vi "HandsOnEmulatedHardware.vi"() -> ()   [LabVIEW 2024]
doc: "DESCRIPTION\nHands On Emulated VISA Hardware\n\nVERSION\nD1:04\nDIs are inverted when compared to hardware - corrected\nRemoved Obsolete GET and SET commands\n20 Oct 2023\n\nD1:03\nMade compatible with CTI-VISA - PWM still to do \n13 Sept 2023\n\nD1:02\nAdded copy VISA REf to clipboard\n28 Jun 2023\n\nTemplate D2:01\nMade lighter and simpler\n14-04-2020"
uses:
  SubVIs/Controls/SetupModeState.ctl
  <vilib>/event_ctls.llb/eventsource.ctl
  SubVIs/Controls/DisplayQCommand.ctl
  SubVIs/Controls/DisplayMessage.ctl
  SubVIs/Controls/Transition.ctl
  SubVIs/utilities/Error/ErrorCommand.ctl
  SubVIs/Controls/QueueCommand.ctl
  SubVIs/Controls/Tab.ctl
  SubVIs/Controls/StateMessage.ctl
  SubVIs/Error/ErrorMessage.ctl
  SubVIs/Controls/Analogs.ctl
  SubVIs/Controls/DigitalOuts.ctl
  SubVIs/Globals/HandsOnGlobals.vi
panel:
  in  "Source":T1 items=["LabVIEW UI"=0, "ActiveX"=1, "User Event"=25]
  out "ErrorHandlingLoop":i32
  out "StateMachineLoop":i32
  out "Version":string="D1:04"
  out "Time":string
  out "UILoop":i32
  out "EventLoop":i32
  in  "Main Screen Tabs":enum32{"Main Screen"}(tab)
  out "Tab Control":T2(tab)
  out "PWMFreq":dbl
  out "PWMDuty":dbl
  out "PWM":dynamicdata(graph)
  in  "Copy":bool
  out "DO4":bool
  out "DO3":bool
  out "DO1":bool
  out "DO2":bool
  in  "DI 1":bool
  in  "DI 2":bool
  in  "DI 3":bool
  out "SCPI Return":string
  out "SCPI":string
  out "BEEP":bool
  in  "AI2":u16(knob) scale=0.0..4096.0
  in  "AI1":u16(knob) caption="Analog Input 1" scale=0.0..4096.0
  in  "DI 4":bool
  out "ConfigdB path":path
  out "Host IP":string="192.168.10.123"
  out "Port":u16=6340
  in  "Home Button":bool
  in  "ErrorLog":bool
  in  "Clear Alarm":bool
  in  "ErrorLog":i32(listbox)
  out "Error":string
  out "ErrorIndicator":bool
  out "State":T3=enum."Connecting"
  in  "ViewError":bool
  out "Status":string
  in  "Start":bool
  in  "exit":bool
  # "Hands On Emulator"
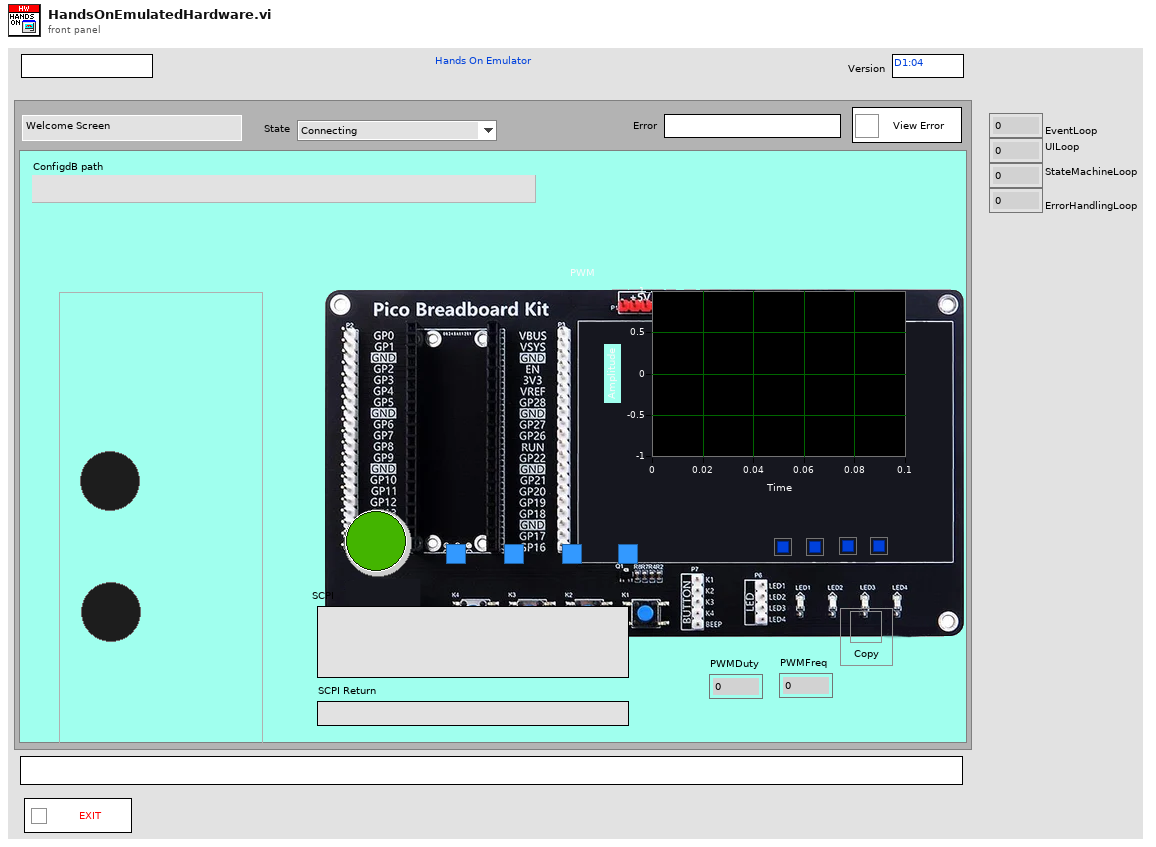
[diagram p1: front panel]
types:
  T1 = typedef "eventsource.ctl" = u32
  T2 = enum32{"Welcome Screen", "Eng Set Up", "Oppo Run Screen", "Eng Run Screen", "Test Report Screen", "Error"}
  T3 = typedef "SetupModeState.ctl" = enum16{"No State - Error", "Connecting", "Running", "Erroring", "Exiting"}
  T4 = typedef "DisplayQCommand.ctl" = enum16{"No Command - Error", "Initialise", "Get Q Reference", "Add Item to Bottom", "Add Item to Top", "Flush Q", "Dequeue", "Peek Next Element", "Close"}
  T5 = typedef "ErrorCommand.ctl" = enum16{"No Command - Error", "Set to Dev Mode", "Set To Released Mode", "Set Error", "Log Error", "Throw Error", "Log & Throw Error", "Set Error Timed"}
  T6 = typedef "QueueCommand.ctl" = enum16{"No Command - Error", "Initialise", "Add to Bottom", "Add To Top", "Get Ref", "Close"}
  T7 = enum32{"invalid app kind", "Development System", "Run Time System", "Student Edition", "Embedded LabVIEW", "Evaluation", "Custom"}
  T8 = typedef "DisplayMessage.ctl" = enum16{"No Message - Ignore", "Display Message", "Set Tab", "Set Status", "Add Error Message", "Clear Error History", "Generate Error", "Set Idling Display", "Set Running Display", "Set DO1", "Set DO2", "Set DO3", "Set DO4", "Set AI1", "Set BEEP", "Update SCPI Return", "Clear SCPI", "Reset Screen", "Set PWM Duty", "Set PWM Freq", "Stop"}
  T9 = typedef "ErrorMessage.ctl" = enum16{"No Message - Ignore", "Display Message", "Stop"}
  T10 = typedef "StateMessage.ctl" = cluster{"Transition":T11, "variant":variant}
  T11 = typedef "Transition.ctl" = enum16{"No Transition - Error", "Initialise", "Connected", "Timed Out", "Disconnected", "Message Rxd", "Generate Error", "Start", "Stop", "Exit"}
  T12 = typedef "Tab.ctl" = enum32{"Welcome Screen", "Eng Set Up", "Oppo Run Screen", "Eng Run Screen", "Test Report Screen", "Error"}
  T13 = typedef "DigitalOuts.ctl" = cluster{"DO1":bool, "DO2":bool, "DO3":bool, "DO4":bool, "BEEP":bool}
  T14 = typedef "Analogs.ctl" = cluster{"AI1":u16, "AI2":u16}
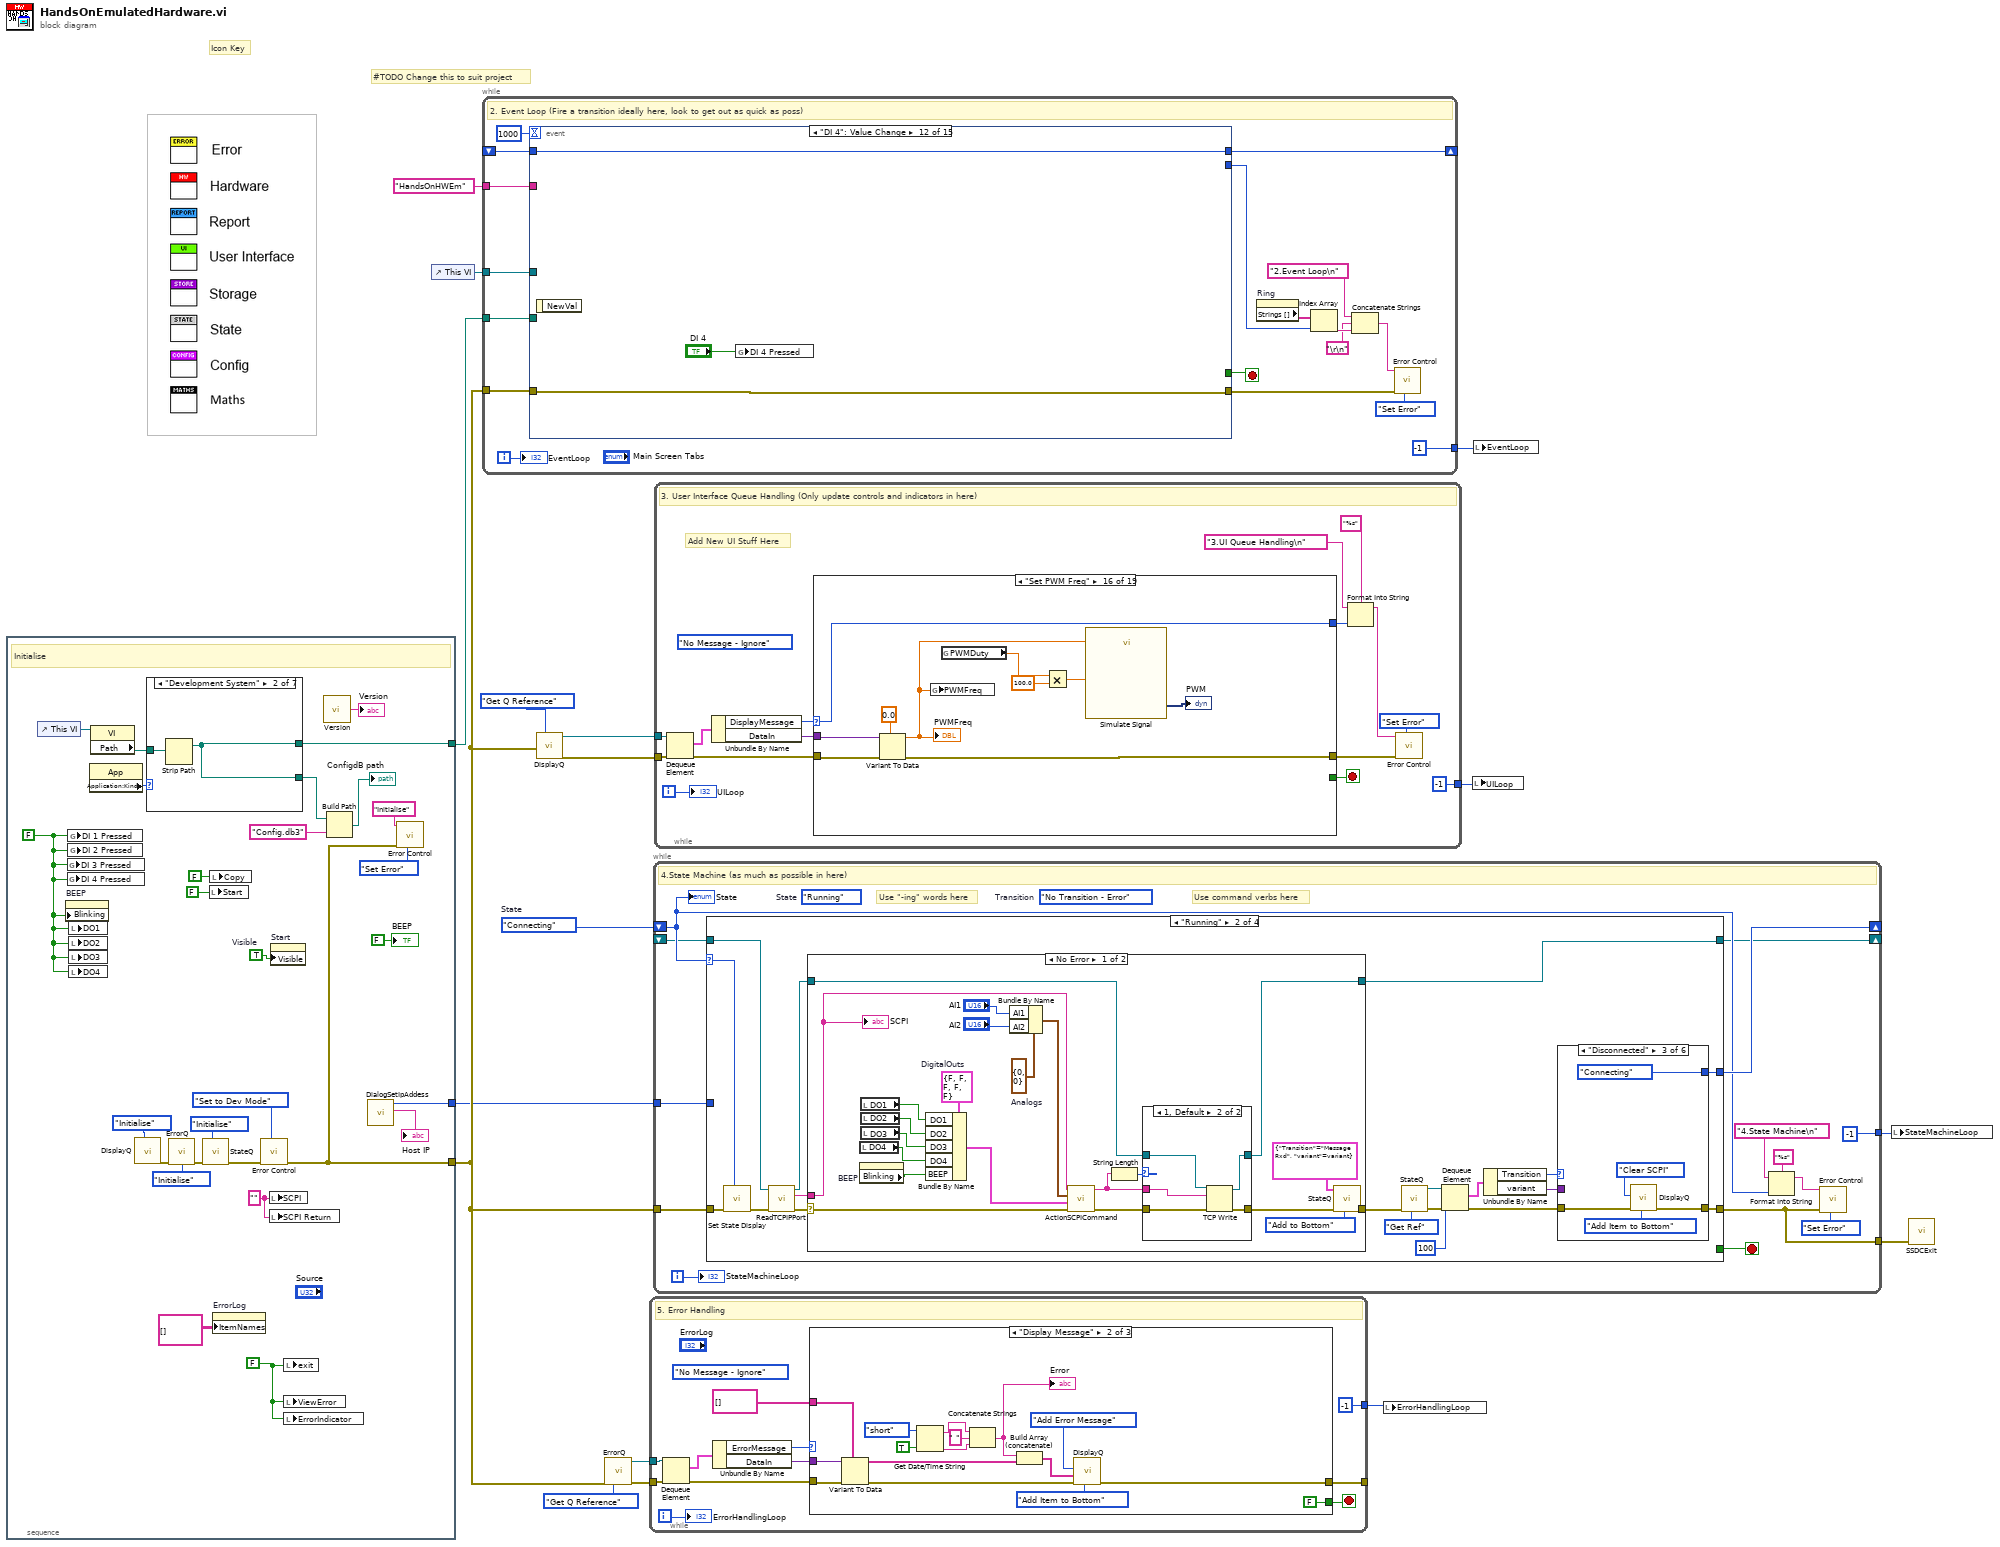
[diagram p0: block diagram]
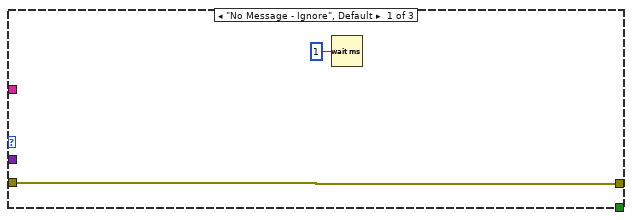
[diagram p2: hidden frame]
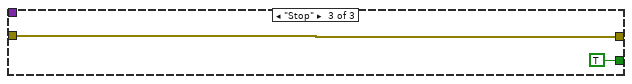
[diagram p3: hidden frame]
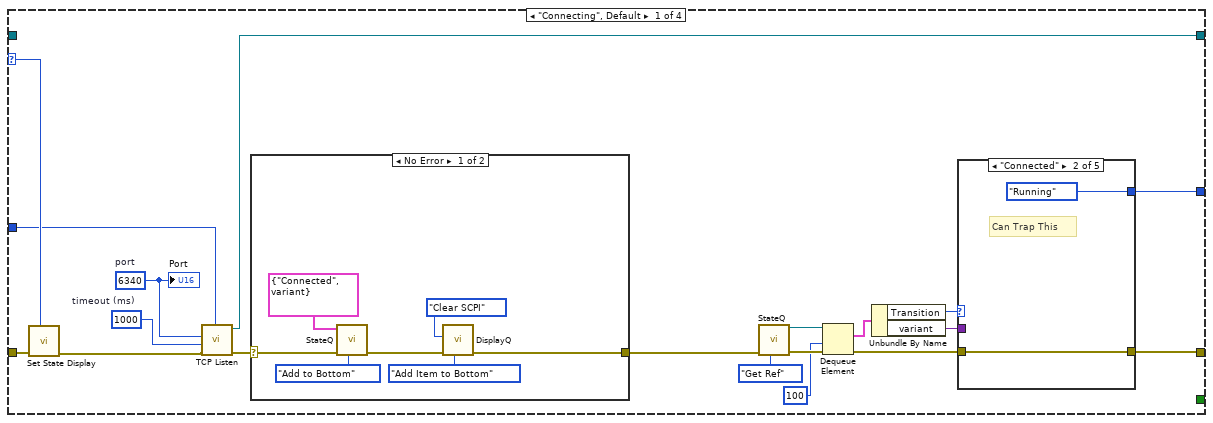
[diagram p4: hidden frame]
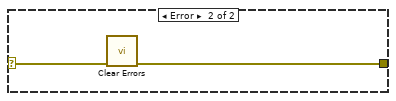
[diagram p5: hidden frame]
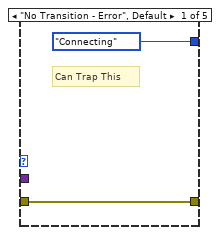
[diagram p6: hidden frame]
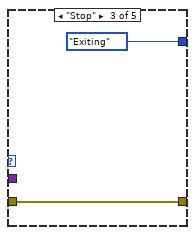
[diagram p7: hidden frame]
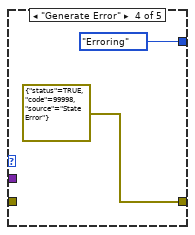
[diagram p8: hidden frame]
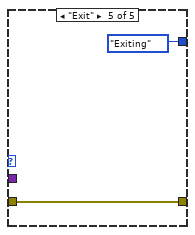
[diagram p9: hidden frame]
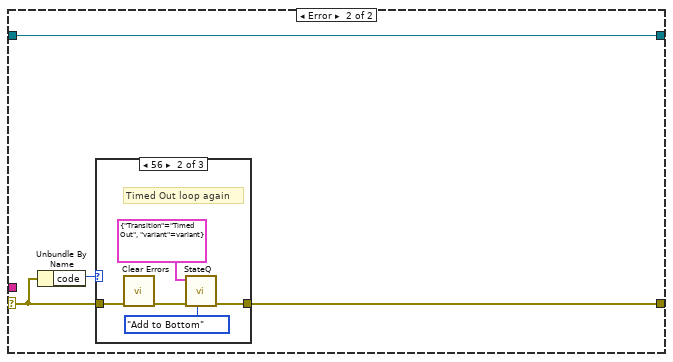
[diagram p11: hidden frame]
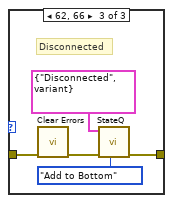
[diagram p13: hidden frame]
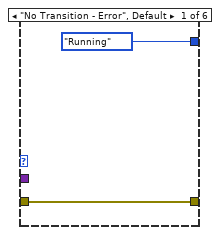
[diagram p14: hidden frame]
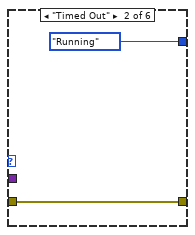
[diagram p15: hidden frame]
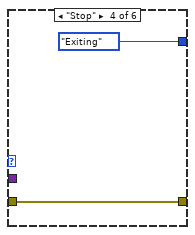
[diagram p16: hidden frame]
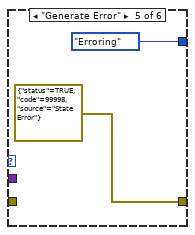
[diagram p17: hidden frame]
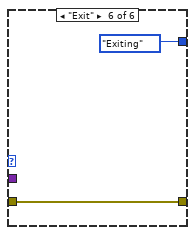
[diagram p18: hidden frame]
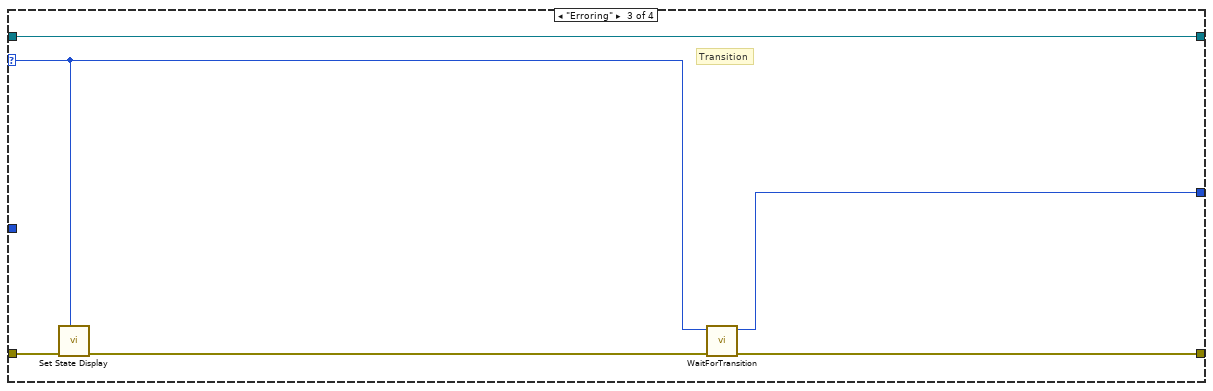
[diagram p19: hidden frame]
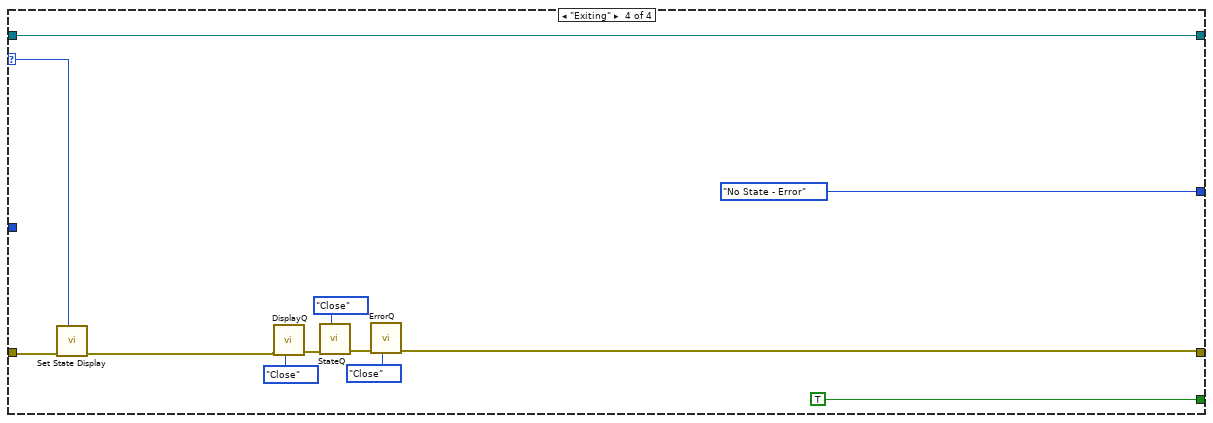
[diagram p20: hidden frame]
diagram:
  w17 = SetupModeState."Connecting"  # State
  # "#TODO Change this to suit project"
  # "Icon Key"
  n1 = stacked-sequence "1. Initialisation" {
    tunnel: [w18] -> w3
    tunnel: [w31] -> w11
    tunnel: [w20] -> w1
    frame #0 {
      w22 = "" ("SCPI")
      w23 = FALSE ("DI 1 Pressed")
      w25 = TRUE  # Visible
      w29 = FALSE ("Stopped")
      # "Initialise"
      n2 = control-ref of="This VI"() -> (w41:refnum<vi>)
      n3 = property on="BEEP" class="Bool (strict)"("Blinking"=w23) -> ()  [unwired: 2 in, 2 out]
      n4 = global write "HandsOnGlobals.vi" "DI 3 Pressed"(w23) -> ()
      n5 = global write "HandsOnGlobals.vi" "DI 4 Pressed"(w23) -> ()
      n6 = global write "HandsOnGlobals.vi" "DI 1 Pressed"(w23) -> ()
      n7 = global write "HandsOnGlobals.vi" "DI 2 Pressed"(w23) -> ()
      n8 = local write "DO1"(w23) -> ()
      n9 = local write "DO2"(w23) -> ()
      n10 = local write "DO3"(w23) -> ()
      n11 = local write "DO4"(w23) -> ()
      n12 = property class="App"() -> ("Application:Kind"=w40:T7)  [unwired: 2 in, 2 out]
      n13 = property class="VI"(reference=w41) -> ("Path"=w42:path)  [unwired: 1 in, 2 out]
      n14 = call "DisplayQ.vi"("command"=DisplayQCommand."Initialise") -> ("error out"=w35:errorcluster)  [unwired: 4 in, 3 out]
      n15 = case shown="\"Development System\"" w40 {
        tunnel: w42 -> [w46 w48 w52 w55 w57 w59 w61]
        tunnel: [w46 w47 w51 w54 w56 w58 w60] -> w32
        tunnel: [w46 w47 w49 w54 w56 w58 w60] -> w31
        frame "invalid app kind", Default {
        }
        frame "Development System" {
          n16 = Strip Path(path=w48) -> (stripped path=w47:path)  [unwired: 1 out]
        }
        frame "Run Time System" {
          n17 = Strip Path(path=w52) -> (stripped path=w53:path)  [unwired: 1 out]
          n18 = Strip Path(path=w53) -> (stripped path=w49:path)  [unwired: 1 out]
          n19 = Build Path(base path=w49, name or relative path="data") -> (appended path=w51:path)
        }
        frame "Student Edition" {
          n20 = Strip Path(path=w55) -> (stripped path=w54:path)  [unwired: 1 out]
        }
        frame "Embedded LabVIEW" {
          n21 = Strip Path(path=w57) -> (stripped path=w56:path)  [unwired: 1 out]
        }
        frame "Evaluation" {
          n22 = Strip Path(path=w59) -> (stripped path=w58:path)  [unwired: 1 out]
        }
        frame "Custom" {
          n23 = Strip Path(path=w61) -> (stripped path=w60:path)  [unwired: 1 out]
        }
      }
      n24 = call "ErrorQ.vi"("command"=DisplayQCommand."Initialise", "error in (no error)"=w35) -> ("error out"=w36:errorcluster)  [unwired: 3 in, 3 out]
      n25 = call "StateQ.vi"("QueueCommand"=QueueCommand."Initialise", "error in (no error)"=w36) -> ("error out"=w27:errorcluster)  [unwired: 5 in, 1 out]
      n26 = local write "Start"(FALSE ("Start")) -> ()
      n27 = local write "Copy"(FALSE ("Copy")) -> ()
      n28 = property on="ErrorLog" class="MCListbox (strict)"("ItemNames"=string[][] [] ("Item Names")) -> ()  [unwired: 2 in, 2 out]
      n29 = call "Error Control.vi"("Command"=ErrorCommand."Set to Dev Mode", "error in (no error)"=w27) -> ("error out"=w18:errorcluster)  [unwired: 6 in]
      n30 = local write "SCPI"(w22) -> ()
      n31 = local write "SCPI Return"(w22) -> ()
      n32 = property on="Start" class="Bool (strict)"("Visible"=w25) -> ()  [unwired: 2 in, 2 out]
      n33 = local write "exit"(w29) -> ()
      n34 = local write "ViewError"(w29) -> ()
      n35 = local write "ErrorIndicator"(w29) -> ()
      n36 = call "Version.vi"() -> ("Version"=→"Version":string)  [unwired: 5 in]
      n37 = Build Path(base path=w32, name or relative path="Config.db3") -> (appended path=→"ConfigdB path":path)
      n38 = call "DialogSetIpAddess.vi"() -> ("Network"=→"Host IP":string, "NetAddress"=w20:u32)  [unwired: 9 in, 1 out]
      n39 = call "Error Control.vi"("Command"=ErrorCommand."Set Error", "error in (no error)"=w18, "Source"="Initialise") -> ()  [unwired: 5 in, 1 out]
      "BEEP" <- FALSE ("DOFlash")
    }
  }
  n40 = control-ref of="This VI"() -> (w16:refnum<vi>)
  n41 = while "2. Event Loop" {
    tunnel: w3 -> [w76]
    shift-right: [w71] -> _
    shift-left: _ -> [w70]
    tunnel: w16 -> [w65]
    tunnel: [-1 ("ErrorHandlingLoop")] -> w12
    tunnel: w11 -> [w63]
    tunnel: "HandsOnHWEm" ("name or relative path") -> [w62]
    i -> [w79]
    stop <- w78 stop-if-true
    # "2. Event Loop (Fire a transition ideally here, look to get out as quick as poss)"
    n42 = event shown="[11] \"DI 4\": Value Change" {
      selector: _ -> [_ _ _ _ _ _ _ _ _ _ _ _ _ _ _]
      dyn-events: _ -> [_ _ _ _ _ _ _ _ _ _ _ _ _ _ _]
      timeout: 1000 -> [_ _ _ _ _ _ _ _ _ _ _ _ _ _ _]
      tunnel: [_ _ FALSE ("STOP?") _ TRUE ("STOP?") _ w144 _ _ _ _ _ _ _ _] -> w78
      tunnel: w76 -> [_ w89 w102 _ _ w127 w140 w160 w176 w187 _ w208 w211 w214 w217]
      tunnel: [_ w90 w102 _ _ w126 w139 w159 w175 w186 _ w208 w211 w214 w217] -> w74
      tunnel: [w81 _ w101 w109 w112 w131 w142 w154 w174 w182 w204 _ _ _ _] -> w72
      tunnel: [w80 w91 w100 w108 w111 w130 w143 w155 w173 w183 w205 w209 w212 w215 w218] -> w71
      tunnel: w70 -> [w80 w91 w100 w108 w111 w130 w143 _ w173 w183 w205 w209 w212 w215 w218]
      tunnel: w65 -> [_ _ _ _ _ _ w141 _ _ _ w203 _ _ _ _]
      tunnel: w63 -> [_ _ _ _ _ _ w138 _ _ _ _ _ _ _ _]
      tunnel: w62 -> [_ _ _ _ _ _ _ _ _ _ _ _ _ _ _]
      event Timeout {
        n43 = event-data() -> ("Source"=w81:T1)  [unwired: 1 in]
        n44 = Get Date/Time String(want seconds? (F)=TRUE) -> (date string=w85:string, time string=w84:string)  [unwired: 2 in]
        n45 = Concatenate Strings(w85, " " ("string"), w84) -> (→"Time":string)
      }
      event "Copy": Value Change {
        n46 = event-data() -> ()  [unwired: 1 in, 6 out]
        n47 = case shown="False" "Copy" {
          tunnel: [w93 w95] -> w90
          tunnel: w89 -> [w93 w94]
          tunnel: [FALSE _] -> w87
          frame False {
          }
          frame True {
            n48 = local read "Host IP"() -> (w98:string)
            n49 = local read "Port"() -> (w97:u16)
            n50 = Format Into String(format string="TCPIP0::%s::%d::SOCKET", w98, w97) -> (resulting string=w96:string)  [unwired: 2 in, 1 out]
            n51 = invoke class="App" method="Clipboard.Write"(error in=w94, "Param 0"=w96) -> (error out=w95:errorcluster)  [unwired: 2 in, 3 out]
          }
        }
        n52 = local write "Copy"(w87) -> ()
      }
      event Panel Close? {
        n53 = event-data() -> ("Source"=w101:T1)  [unwired: 1 in]
        n54 = property on="exit" class="Bool (strict)"("Val(Sgnl)"=TRUE ("Value (Signaling)")) -> ()  [unwired: 2 in, 2 out]
        n55 = event-data("Discard?"=TRUE) -> ()  [unwired: 1 in, 1 out]
      }
      event "ErrorLog": Value Change {
        n56 = event-data() -> ("Source"=w109:T1)  [unwired: 1 in, 5 out]
        n57 = case shown="True" "ErrorLog" {
          tunnel: [_ FALSE] -> w106
          frame False {
          }
          frame True {
          }
        }
        n58 = local write "ErrorLog"(w106) -> ()
      }
      event "exit": Value Change {
        n59 = event-data() -> ("Source"=w112:T1)  [unwired: 1 in, 2 out]
        n60 = local write "Start"(FALSE ("Start")) -> ()
        n61 = stacked-sequence {
          tunnel: [_ FALSE] -> w113
          frame #0 {
            n62 = call "StateQ.vi"("QueueCommand"=QueueCommand."Add To Top", "output cluster"=T10 {"Transition"=enum."Exit", "variant"=variant}) -> ("error out"=w120:errorcluster)  [unwired: 5 in, 1 out]
            n63 = call "ErrorQ.vi"("command"=DisplayQCommand."Add Item to Top", "error in (no error)"=w120, "ErrorMessage"=ErrorMessage."Stop") -> ("error out"=w117:errorcluster)  [unwired: 2 in, 3 out]
            n64 = call "DisplayQ.vi"("command"=DisplayQCommand."Add Item to Top", "error in (no error)"=w117, "DisplayMessage"=DisplayMessage."Stop") -> ()  [unwired: 2 in, 4 out]
          }
          frame #1 {
            n65 = Wait (ms)(milliseconds to wait=u32 500) -> ()  [unwired: 1 out]
          }
        }
        n66 = local write "exit"(w113) -> ()
      }
      event "Start": Value Change {
        n67 = event-data() -> ("Source"=w131:T1)  [unwired: 1 in, 5 out]
        n68 = case shown="True" "Start" {
          tunnel: [_ FALSE ("Start")] -> w128
          tunnel: w127 -> [w132 w134]
          tunnel: [w132 w133] -> w126
          frame False {
          }
          frame True {
            n69 = call "StateQ.vi"("QueueCommand"=QueueCommand."Add To Top", "error in (no error)"=w134, "output cluster"=T10 {"Transition"=enum."Start", "variant"=variant}) -> ("error out"=w133:errorcluster)  [unwired: 4 in, 1 out]
          }
        }
        n70 = local write "Start"(w128) -> ()
      }
      event Menu Selection (User) {
        n71 = event-data() -> ("Source"=w142:T1, "ItemTag"=w145:string)  [unwired: 1 in]
        n72 = case shown="\"Configuration\"" w145 {
          tunnel: [_ FALSE _ _] -> w144
          tunnel: w141 -> [_ _ _ w153]
          tunnel: w140 -> [w146 w147 w150 w151]
          tunnel: [w146 w147 w150 w151] -> w139
          tunnel: w138 -> [_ _ _ _]
          frame "False", Default {
          }
          frame "Exit" {
            n73 = property on="exit" class="Bool (strict)"("Val(Sgnl)"=TRUE ("Value (Signaling)")) -> ()  [unwired: 2 in, 2 out]
          }
          frame "Configuration" {
          }
          frame "About" {
            n74 = property class="VI"(reference=w153) -> ("Description"=w152:string)  [unwired: 1 in, 2 out]
            n75 = call "AboutScreen.vi"("Version Info. In"=w152) -> ()  [unwired: 11 in]
          }
        }
      }
      event "ViewError": Value Change {
        n76 = event-data() -> ("Source"=w154:T1)  [unwired: 1 in]
        n77 = local read "Tab Control"() -> (w156:T2)
        n78 = case shown="True" "ViewError" {
          tunnel: w160 -> [w163 w167]
          tunnel: [w163 w166] -> w159
          tunnel: [FALSE FALSE] -> w157
          tunnel: w156 -> [w161 w164]
          tunnel: [w161 w164] -> w155
          frame False {
          }
          frame True {
            n79 = call "DisplayQ.vi"("command"=DisplayQCommand."Add Item to Bottom", "error in (no error)"=w167, "DataIn"=Tab."Error" ("Tab Control"), "DisplayMessage"=DisplayMessage."Set Tab") -> ("error out"=w166:errorcluster)  [unwired: 1 in, 3 out]
          }
        }
        n80 = local write "ViewError"(w157) -> ()
      }
      event "Clear Alarm": Value Change {
        n81 = event-data() -> ("Source"=w174:T1)  [unwired: 1 in]
        n82 = case shown="False" "Clear Alarm" {
          tunnel: w176 -> [w178 w180]
          tunnel: [w178 w180] -> w175
          tunnel: [FALSE FALSE] -> w171
          frame False {
          }
          frame True {
            n83 = local write "ErrorIndicator"(FALSE ("ErrorIndicator")) -> ()
          }
        }
        n84 = local write "Clear Alarm"(w171) -> ()
      }
      event "Home Button": Value Change {
        n85 = event-data() -> ("Source"=w182:T1)  [unwired: 1 in]
        n86 = case shown="True" "Home Button" {
          tunnel: w187 -> [w189 w194]
          tunnel: [w189 w193] -> w186
          tunnel: [FALSE FALSE] -> w185
          tunnel: w183 -> [_ w191]
          frame False {
          }
          frame True {
            n87 = case shown="\"Error\"" w191 {
              tunnel: [Tab."Welcome Screen" ("Tab Control") Tab."Oppo Run Screen" ("Tab Control") Tab."Eng Run Screen" ("Tab Control") Tab."Test Report Screen" ("Tab Control") Tab."Error" ("Tab Control") Tab."Eng Run Screen" ("Tab Control")] -> w190
              frame "Welcome Screen" {
              }
              frame "Oppo Run Screen" {
              }
              frame "Eng Run Screen" {
              }
              frame "Test Report Screen" {
              }
              frame "Error" {
              }
              frame "Eng Set Up" {
              }
            }
            n88 = call "DisplayQ.vi"("command"=DisplayQCommand."Add Item to Bottom", "error in (no error)"=w194, "DataIn"=w190, "DisplayMessage"=DisplayMessage."Set Tab") -> ("error out"=w193:errorcluster)  [unwired: 1 in, 3 out]
          }
        }
        n89 = local write "Home Button"(w185) -> ()
      }
      event "Version": Mouse Down {
        n90 = event-data() -> ("Source"=w204:T1)  [unwired: 1 in]
        n91 = property class="VI"(reference=w203) -> ("Description"=w206:string)  [unwired: 1 in, 2 out]
        n92 = call "VIDescription.vi"("VersionData In"=w206) -> ()  [unwired: 10 in, 1 out]
      }
      event "DI 4": Value Change {
        n93 = event-data() -> ()  [unwired: 1 in, 1 out]
        n94 = global write "HandsOnGlobals.vi" "DI 4 Pressed"("DI 4") -> ()
      }
      event "DI 3": Value Change {
        n95 = event-data() -> ()  [unwired: 1 in, 1 out]
        n96 = global write "HandsOnGlobals.vi" "DI 3 Pressed"("DI 3") -> ()
      }
      event "DI 2": Value Change {
        n97 = event-data() -> ()  [unwired: 1 in, 1 out]
        n98 = global write "HandsOnGlobals.vi" "DI 2 Pressed"("DI 2") -> ()
      }
      event "DI 1": Value Change {
        n99 = event-data() -> ()  [unwired: 1 in, 1 out]
        n100 = global write "HandsOnGlobals.vi" "DI 1 Pressed"("DI 1") -> ()
      }
    }
    n101 = property on="Ring" class="Ring (strict)"() -> ("Strings []"=w73:string[])  [unwired: 2 in, 2 out]
    n102 = Index Array(array=w73, index=w72) -> (element=w69:string)
    n103 = Concatenate Strings("2.Event Loop\n", "\r\n", w69) -> (w68:string)
    n104 = call "Error Control.vi"("Command"=ErrorCommand."Set Error", "error in (no error)"=w74, "Source"=w68) -> ()  [unwired: 5 in, 1 out]
    "EventLoop" <- w79
  }
  n105 = call "DisplayQ.vi"("command"=DisplayQCommand."Get Q Reference", "error in (no error)"=w3) -> ("error out"=w5:errorcluster, "queue out"=w6:refnum<queue>)  [unwired: 3 in, 2 out]
  n106 = call "ErrorQ.vi"("command"=DisplayQCommand."Get Q Reference", "error in (no error)"=w3) -> ("error out"=w8:errorcluster, "queue out"=w9:refnum<queue>)  [unwired: 3 in, 2 out]
  n107 = while {
    tunnel: w8 -> [w229]
    tunnel: w9 -> [w228]
    tunnel: [w220] -> _
    tunnel: [-1 ("ErrorHandlingLoop")] -> w15
    i -> [w222]
    stop <- w223 stop-if-true
    (unwired) DisplayMessage."No Message - Ignore" ("DisplayMessage")
    # "5. Error Handling"
    n108 = Dequeue Element(queue=w228, error in (no error)=w229) -> (element=w227:cluster{"ErrorMessage":T9, "DataIn":variant}, error out=w224:errorcluster)  [unwired: 1 in, 2 out]
    n109 = Unbundle By Name(w227) -> ("ErrorMessage"=w225:T9, "DataIn"=w226:variant)
    n110 = case shown="\"Display Message\"" w225 {
      tunnel: w226 -> [_ w246 _]
      tunnel: w224 -> [w230 w245 w249]
      tunnel: [w230 w236 w249] -> w220
      tunnel: [_ FALSE ("STOP?") TRUE ("STOP?")] -> w223
      tunnel: string[] [] -> [_ w244 _]
      frame "No Message - Ignore", Default {
        n111 = Wait (ms)(milliseconds to wait=u32 1) -> ()  [unwired: 1 out]
      }
      frame "Display Message" {
        n112 = Variant To Data(error in=w245, type=w244, Variant=w246) -> (data=w238:string[], error out=w237:errorcluster)
        n113 = Get Date/Time String(date format (0)=enum16{"short", "long", "abbreviated"}."short", want seconds? (F)=TRUE) -> (date string=w241:string, time string=w240:string)  [unwired: 1 in]
        n114 = Concatenate Strings(w241, " " ("string"), w240) -> (w232:string)
        "Error" <- w232
        n115 = Build Array (concatenate)(w232, w238) -> (w233:string[])
        n116 = call "DisplayQ.vi"("command"=DisplayQCommand."Add Item to Bottom", "error in (no error)"=w237, "DataIn"=w233, "DisplayMessage"=DisplayMessage."Add Error Message") -> ("error out"=w236:errorcluster)  [unwired: 1 in, 3 out]
      }
      frame "Stop" {
      }
    }
    "ErrorHandlingLoop" <- w222
  }
  n117 = while {
    shift-right: [w261] -> _
    shift-left: w17 -> [w258]
    tunnel: w3 -> [w262]
    tunnel: [-1 ("ErrorHandlingLoop")] -> w14
    shift-right: [w253] -> _
    shift-left: _ -> [w252]
    tunnel: [w251] -> w2
    tunnel: w1 -> [w250]
    i -> [w260]
    stop <- w263 stop-if-true
    (unwired) SetupModeState."Running"  # State
    (unwired) Transition."No Transition - Error"  # Transition
    # "Use command verbs here"
    # "Use \"-ing\" words here"
    # "4.State Machine (as much as possible in here)"
    n118 = case shown="\"Running\"" w258 {
      selector: w258 -> [w265 w319 w381 w394]
      tunnel: [_ _ _ TRUE] -> w263
      tunnel: w262 -> [w267 w320 w385 w395]
      tunnel: [w273 w311 w384 SetupModeState."No State - Error" ("State 2")] -> w261
      tunnel: [w275 w312 w383 w386] -> w251
      tunnel: [w268 w302 w380 w393] -> w253
      tunnel: w252 -> [_ w309 w380 w393]
      tunnel: w250 -> [w264 _ _ _]
      frame "Connecting", Default {
        w271 = u16 6340  # port
        w272 = 1000  # timeout (ms)
        n119 = call "Set State Display.vi"("State"=w265, "error in (no error)"=w267) -> ("error out"=w266:errorcluster)  [unwired: 6 in]
        n120 = call <vilib>:"TCP Listen.vi"("net address"=w264, "error in (no error)"=w266, "timeout ms (wait forever: -1)"=w272, "port"=w271) -> ("error out"=w270:errorcluster, "connection ID"=w268:refnum<k5>)  [unwired: 3 in, 3 out]
        n121 = case shown="No Error" w270 {
          selector: w270 -> [w287 w290]
          tunnel: [w283 w291] -> w269
          frame No Error {
            n122 = call "StateQ.vi"("QueueCommand"=QueueCommand."Add to Bottom", "error in (no error)"=w287, "output cluster"=T10 {"Transition"=enum."Connected", "variant"=variant}) -> ("error out"=w285:errorcluster)  [unwired: 4 in, 1 out]
            n123 = call "DisplayQ.vi"("command"=DisplayQCommand."Add Item to Bottom", "error in (no error)"=w285, "DisplayMessage"=DisplayMessage."Clear SCPI") -> ("error out"=w283:errorcluster)  [unwired: 2 in, 3 out]
          }
          frame Error {
            n124 = call <vilib>:"Clear Errors.vi"("error in (no error)"=w290) -> ("error out"=w291:errorcluster)  [unwired: 5 in, 1 out]
          }
        }
        n125 = call "StateQ.vi"("QueueCommand"=QueueCommand."Get Ref", "error in (no error)"=w269) -> ("error out"=w280:errorcluster, "queue out"=w279:refnum<queue>)  [unwired: 5 in]
        n126 = Dequeue Element(queue=w279, timeout in ms (-1)=100, error in (no error)=w280) -> (element=w282:T10, error out=w278:errorcluster)  [unwired: 2 out]
        n127 = Unbundle By Name(w282) -> ("Transition"=w277:T11, "variant"=w276:variant)
        n128 = case shown="\"Connected\"" w277 {
          tunnel: [SetupModeState."Connecting" ("State 2") SetupModeState."Running" ("State 2") SetupModeState."Exiting" ("State 2") SetupModeState."Erroring" ("State 2") SetupModeState."Exiting" ("State 2")] -> w273
          tunnel: w278 -> [w292 w294 w296 _ w300]
          tunnel: [w292 w294 w296 errorcluster {"status"=TRUE, "code"=99998, "source"="State Error"} ("error out") w300] -> w275
          tunnel: w276 -> [_ _ _ _ _]
          frame "No Transition - Error", Default {
            # "Can Trap This"
          }
          frame "Connected" {
            # "Can Trap This"
          }
          frame "Stop" {
          }
          frame "Generate Error" {
          }
          frame "Exit" {
          }
        }
        "Port" <- w271
      }
      frame "Running" {
        n129 = call "Set State Display.vi"("State"=w319, "error in (no error)"=w320) -> ("error out"=w308:errorcluster)  [unwired: 6 in]
        n130 = call "ReadTCPIPPort.vi"("error in (no error)"=w308, "TCP Network Connection in"=w309) -> ("error out"=w307:errorcluster, "data out"=w306:string, "TCP Network Connection out"=w303:refnum<k5>)  [unwired: 7 in]
        n131 = case shown="No Error" w307 {
          selector: w307 -> [w328 w353]
          tunnel: w306 -> [w327 _]
          tunnel: [w341 w350] -> w305
          tunnel: w303 -> [w322 w351]
          tunnel: [w321 w351] -> w302
          frame No Error {
            w329 = T13 {"DO1"=FALSE, "DO2"=FALSE, "DO3"=FALSE, "DO4"=FALSE, "BEEP"=FALSE}  # DigitalOuts
            w330 = T14 {"AI1"=0, "AI2"=0}  # Analogs
            n132 = local read "DO4"() -> (w334:bool)
            n133 = property on="BEEP" class="Bool (strict)"() -> ("Blinking"=w331:bool)  [unwired: 2 in, 2 out]
            n134 = local read "DO1"() -> (w339:bool)
            n135 = local read "DO2"() -> (w336:bool)
            n136 = local read "DO3"() -> (w335:bool)
            n137 = Bundle By Name(cluster=w329, "DO1"=w339, "DO2"=w336, "DO3"=w335, "DO4"=w334, "BEEP"=w331) -> (w338:T13)
            n138 = Bundle By Name(cluster=w330, "AI1"="AI1", "AI2"="AI2") -> (w337:T14)
            n139 = call "ActionSCPICommand.vi"("error in (no error)"=w328, "DigitalOuts"=w338, "Analogs"=w337, "SCPI"=w327) -> ("error out"=w326:errorcluster, "OutputMessage"=w323:string)  [unwired: 6 in]
            n140 = String Length(string=w323) -> (length=w325:i32)
            n141 = case shown="1, Default" w325 {
              tunnel: w326 -> [w344 w348]
              tunnel: [w344 w349] -> w324
              tunnel: w323 -> [_ w345]
              tunnel: w322 -> [w343 w347]
              tunnel: [w343 w346] -> w321
              frame 0 {
              }
              frame 1, Default {
                n142 = TCP Write(connection ID=w347, data in=w345, error in (no error)=w348) -> (connection ID out=w346:refnum<k5>, error out=w349:errorcluster)  [unwired: 1 in, 1 out]
              }
            }
            n143 = call "StateQ.vi"("QueueCommand"=QueueCommand."Add to Bottom", "error in (no error)"=w324, "output cluster"=T10 {"Transition"=enum."Message Rxd", "variant"=variant}) -> ("error out"=w341:errorcluster)  [unwired: 4 in, 1 out]
            "SCPI" <- w327
          }
          frame Error {
            n144 = Unbundle By Name(w353) -> ("code"=w352:i32)
            n145 = case shown="56" w352 {
              tunnel: [w354 w358 w364] -> w350
              tunnel: w353 -> [w354 w355 w360]
              frame 0, Default {
                # "Undefined error"
              }
              frame 56 {
                # "Timed Out loop again"
                n146 = call <vilib>:"Clear Errors.vi"("error in (no error)"=w355) -> ("error out"=w356:errorcluster)  [unwired: 5 in, 1 out]
                n147 = call "StateQ.vi"("QueueCommand"=QueueCommand."Add to Bottom", "error in (no error)"=w356, "output cluster"=T10 {"Transition"=enum."Timed Out", "variant"=variant}) -> ("error out"=w358:errorcluster)  [unwired: 4 in, 1 out]
              }
              frame 62, 66 {
                # "Disconnected"
                n148 = call <vilib>:"Clear Errors.vi"("error in (no error)"=w360) -> ("error out"=w361:errorcluster)  [unwired: 5 in, 1 out]
                n149 = call "StateQ.vi"("QueueCommand"=QueueCommand."Add to Bottom", "error in (no error)"=w361, "output cluster"=T10 {"Transition"=enum."Disconnected", "variant"=variant}) -> ("error out"=w364:errorcluster)  [unwired: 4 in, 1 out]
              }
            }
          }
        }
        n150 = call "StateQ.vi"("QueueCommand"=QueueCommand."Get Ref", "error in (no error)"=w305) -> ("error out"=w316:errorcluster, "queue out"=w315:refnum<queue>)  [unwired: 5 in]
        n151 = Dequeue Element(queue=w315, timeout in ms (-1)=100, error in (no error)=w316) -> (element=w318:T10, error out=w314:errorcluster)  [unwired: 2 out]
        n152 = Unbundle By Name(w318) -> ("Transition"=w313:T11, "variant"=w310:variant)
        n153 = case shown="\"Disconnected\"" w313 {
          tunnel: [SetupModeState."Running" ("State 2") SetupModeState."Running" ("State 2") SetupModeState."Connecting" ("State 2") SetupModeState."Exiting" ("State 2") SetupModeState."Erroring" ("State 2") SetupModeState."Exiting" ("State 2")] -> w311
          tunnel: w314 -> [w365 w367 w370 w374 _ w378]
          tunnel: [w365 w367 w369 w374 errorcluster {"status"=TRUE, "code"=99998, "source"="State Error"} ("error out") w378] -> w312
          tunnel: w310 -> [_ _ _ _ _ _]
          frame "No Transition - Error", Default {
          }
          frame "Timed Out" {
          }
          frame "Disconnected" {
            n154 = call "DisplayQ.vi"("command"=DisplayQCommand."Add Item to Bottom", "error in (no error)"=w370, "DisplayMessage"=DisplayMessage."Clear SCPI") -> ("error out"=w369:errorcluster)  [unwired: 2 in, 3 out]
          }
          frame "Stop" {
          }
          frame "Generate Error" {
          }
          frame "Exit" {
          }
        }
      }
      frame "Erroring" {
        # "Transition"
        n155 = call "Set State Display.vi"("State"=w381, "error in (no error)"=w385) -> ("error out"=w382:errorcluster)  [unwired: 6 in]
        n156 = call "WaitForTransition.vi"("error in (no error)"=w382, "State"=w381) -> ("error out"=w383:errorcluster, "StateOut"=w384:T3)  [unwired: 4 in]
      }
      frame "Exiting" {
        n157 = call "Set State Display.vi"("State"=w394, "error in (no error)"=w395) -> ("error out"=w387:errorcluster)  [unwired: 6 in]
        n158 = call "DisplayQ.vi"("command"=DisplayQCommand."Close", "error in (no error)"=w387) -> ("error out"=w389:errorcluster)  [unwired: 3 in, 3 out]
        n159 = call "StateQ.vi"("QueueCommand"=QueueCommand."Close", "error in (no error)"=w389) -> ("error out"=w391:errorcluster)  [unwired: 5 in, 1 out]
        n160 = call "ErrorQ.vi"("command"=DisplayQCommand."Close", "error in (no error)"=w391) -> ("error out"=w386:errorcluster)  [unwired: 3 in, 3 out]
      }
    }
    n161 = Format Into String(format string="%s", initial string="4.State Machine\n", w258) -> (resulting string=w257:string)  [unwired: 1 in, 1 out]
    n162 = call "Error Control.vi"("Command"=ErrorCommand."Set Error", "error in (no error)"=w251, "Source"=w257) -> ()  [unwired: 5 in, 1 out]
    "StateMachineLoop" <- w260
    "State" <- w258
  }
  n163 = while "3. User Interface Queue Handling" {
    tunnel: w5 -> [w412]
    tunnel: w6 -> [w411]
    tunnel: [-1 ("ErrorHandlingLoop")] -> w13
    i -> [w404]
    stop <- w405 stop-if-true
    (unwired) DisplayMessage."No Message - Ignore" ("DisplayMessage")
    # "Add New UI Stuff Here"
    # "3. User Interface Queue Handling (Only update controls and indicators in here)"
    n164 = Dequeue Element(queue=w411, error in (no error)=w412) -> (element=w410:cluster{"DisplayMessage":T8, "DataIn":variant}, error out=w407:errorcluster)  [unwired: 1 in, 2 out]
    n165 = Unbundle By Name(w410) -> ("DisplayMessage"=w408:T8, "DataIn"=w409:variant)
    n166 = case shown="\"Set PWM Freq\"" w408 {
      selector: w408 -> [w413 w417 w424 w433 w440 w442 w445 w448 w451 w457 w463 w469 w475 w484 w494 w504 w506 w508 w511]
      tunnel: w409 -> [_ w421 w427 w436 _ _ _ _ w454 w460 w466 w472 w478 w481 w491 w501 _ _ _]
      tunnel: w407 -> [w414 w419 w425 w435 w439 _ w444 w447 w453 w459 w465 w471 w477 w482 w492 w502 w507 w510 w513]
      tunnel: [w414 w418 w422 w434 w439 errorcluster {"status"=TRUE, "code"=99997, "source"="UI Error"} ("error out") w444 w447 w452 w458 w464 w470 w476 w483 w493 w503 w507 w510 w513] -> w398
      tunnel: [_ _ _ _ _ _ _ _ _ _ _ _ _ _ _ _ _ _ TRUE ("STOP?")] -> w405
      tunnel: [w413 w417 w424 w433 w440 w442 w445 w448 w451 w457 w463 w469 w475 w484 w494 w504 w506 w508 w511] -> w403
      frame "No Message - Ignore", Default {
        n167 = Wait (ms)(milliseconds to wait=u32 1) -> ()  [unwired: 1 out]
      }
      frame "Display Message" {
        n168 = Variant To Data(error in=w419, type="" ("data"), Variant=w421) -> (data=→"Status":string, error out=w418:errorcluster)
      }
      frame "Set Tab" {
        n169 = Variant To Data(error in=w425, type=Tab."Eng Run Screen" ("Tab Control"), Variant=w427) -> (data=→"Tab Control":T12, error out=w422:errorcluster)
      }
      frame "Add Error Message" {
        n170 = property on="ErrorLog" class="MCListbox (strict)"() -> ("ItemNames"=w431:string[][])  [unwired: 2 in, 2 out]
        n171 = Variant To Data(error in=w435, type=string[] [], Variant=w436) -> (data=w430:string[], error out=w434:errorcluster)
        n172 = Build Array (concatenate)(w431, w430) -> (w428:string[][])
        n173 = property on="ErrorLog" class="MCListbox (strict)"("ItemNames"=w428) -> ()  [unwired: 2 in, 2 out]
        "ErrorIndicator" <- TRUE ("ErrorIndicator")
      }
      frame "Clear Error History" {
        n174 = property on="ErrorLog" class="MCListbox (strict)"("ItemNames"=string[][] []) -> ()  [unwired: 2 in, 2 out]
        n175 = local write "ErrorIndicator"(FALSE ("ErrorIndicator")) -> ()
      }
      frame "Generate Error" {
      }
      frame "Set Idling Display" {
        w443 = TRUE  # Visible
        n176 = property on="Start" class="Bool (strict)"("Visible"=w443) -> ()  [unwired: 2 in, 2 out]
      }
      frame "Set Running Display" {
        w446 = FALSE  # Visible
        n177 = property on="Start" class="Bool (strict)"("Visible"=w446) -> ()  [unwired: 2 in, 2 out]
      }
      frame "Set DO1" {
        n178 = Variant To Data(error in=w453, type=FALSE, Variant=w454) -> (data=→"DO1":bool, error out=w452:errorcluster)
      }
      frame "Set DO2" {
        n179 = Variant To Data(error in=w459, type=FALSE, Variant=w460) -> (data=→"DO2":bool, error out=w458:errorcluster)
      }
      frame "Set BEEP" {
        n180 = Variant To Data(error in=w465, type=FALSE, Variant=w466) -> (data=w461:bool, error out=w464:errorcluster)
        n181 = property on="BEEP" class="Bool (strict)"("Blinking"=w461) -> ()  [unwired: 2 in, 2 out]
      }
      frame "Set DO3" {
        n182 = Variant To Data(error in=w471, type=FALSE, Variant=w472) -> (data=→"DO3":bool, error out=w470:errorcluster)
      }
      frame "Set DO4" {
        n183 = Variant To Data(error in=w477, type=FALSE, Variant=w478) -> (data=→"DO4":bool, error out=w476:errorcluster)
      }
      frame "Update SCPI Return" {
        n184 = Variant To Data(error in=w482, type="", Variant=w481) -> (data=→"SCPI Return":string, error out=w483:errorcluster)
      }
      frame "Set PWM Duty" {
        n185 = Variant To Data(error in=w492, type=0.0, Variant=w491) -> (data=w489:dbl, error out=w493:errorcluster)
        "PWMDuty" <- w489
        n186 = global write "HandsOnGlobals.vi" "PWMDuty"(w489) -> ()
        n187 = global read "HandsOnGlobals.vi" "PWMFreq"() -> (w488:dbl)
        n188 = Multiply(x=w489, y=100.0) -> (x*y=w486:dbl)
        n189 = call "Simulate Signal2"("Duty Cycle (%)"=w486, "Frequency"=w488) -> ("Square"=w487:dynamicdata)  [unwired: 12 in, 1 out]
        n190 = local write "PWM"(w487) -> ()
      }
      frame "Set PWM Freq" {
        n191 = Variant To Data(error in=w502, type=0.0, Variant=w501) -> (data=w499:dbl, error out=w503:errorcluster)
        "PWMFreq" <- w499
        n192 = global write "HandsOnGlobals.vi" "PWMFreq"(w499) -> ()
        n193 = global read "HandsOnGlobals.vi" "PWMDuty"() -> (w496:dbl)
        n194 = Multiply(x=w496, y=100.0) -> (x*y=w497:dbl)
        n195 = call "Simulate Signal"("Duty Cycle (%)"=w497, "Frequency"=w499) -> ("Square"=→"PWM":dynamicdata)  [unwired: 12 in, 1 out]
      }
      frame "Clear SCPI" {
        w505 = "" ("SCPI")
        n196 = local write "SCPI"(w505) -> ()
        n197 = local write "SCPI Return"(w505) -> ()
      }
      frame "Reset Screen" {
        w509 = FALSE ("DI 1 Pressed")
        n198 = property on="BEEP" class="Bool (strict)"("Blinking"=w509) -> ()  [unwired: 2 in, 2 out]
        n199 = global write "HandsOnGlobals.vi" "DI 3 Pressed"(w509) -> ()
        n200 = global write "HandsOnGlobals.vi" "DI 4 Pressed"(w509) -> ()
        n201 = global write "HandsOnGlobals.vi" "DI 1 Pressed"(w509) -> ()
        n202 = global write "HandsOnGlobals.vi" "DI 2 Pressed"(w509) -> ()
        n203 = local write "DO1"(w509) -> ()
        n204 = local write "DO2"(w509) -> ()
        n205 = local write "DO3"(w509) -> ()
        n206 = local write "DO4"(w509) -> ()
      }
      frame "Stop" {
      }
    }
    n207 = Format Into String(format string="%s", initial string="3.UI Queue Handling\n", w403) -> (resulting string=w402:string)  [unwired: 1 in, 1 out]
    n208 = call "Error Control.vi"("Command"=ErrorCommand."Set Error", "error in (no error)"=w398, "Source"=w402) -> ()  [unwired: 5 in, 1 out]
    "UILoop" <- w404
  }
  n209 = local write "ErrorHandlingLoop"(w15) -> ()
  n210 = local write "UILoop"(w13) -> ()
  n211 = local write "EventLoop"(w12) -> ()
  n212 = local write "StateMachineLoop"(w14) -> ()
  n213 = call "SSDCExit.vi"("error in (no error)"=w2) -> ()  [unwired: 6 in, 1 out]
